vi "top_level.vi"(10 "progress ref":refnum<vi>, 11 "series URL":string) -> (0 "error out":errorcluster, 2 "fetch time":dbl, 3 "seriesInfo":T2)   [LabVIEW 2024]
uses:
  definitions/seriesInfo.ctl
  definitions/issueInfo.ctl
  definitions/creator.ctl
  definitions/character.ctl
  definitions/team.ctl
  definitions/location.ctl
  definitions/concept.ctl
  definitions/thing.ctl
  definitions/storyArc.ctl
  definitions/seriesJSON.ctl
  series_class/series_class.lvclass
  C:/Code/LabVIEW_Projects/applications/ComicVine_API/comic_class/comic_class.lvclass
  series_class/series_class.lvclass/series_class.ctl
  <vilib>/Utility/High Resolution Relative Seconds.vi
  comic_class/comic_class.lvclass
  <vilib>/addons/_JKI.lib/Serialization/JSON/JKI JSON Serialization.lvlib
panel:
  in  "output cluster":T1
  out "issues":T3[](array[typedef])
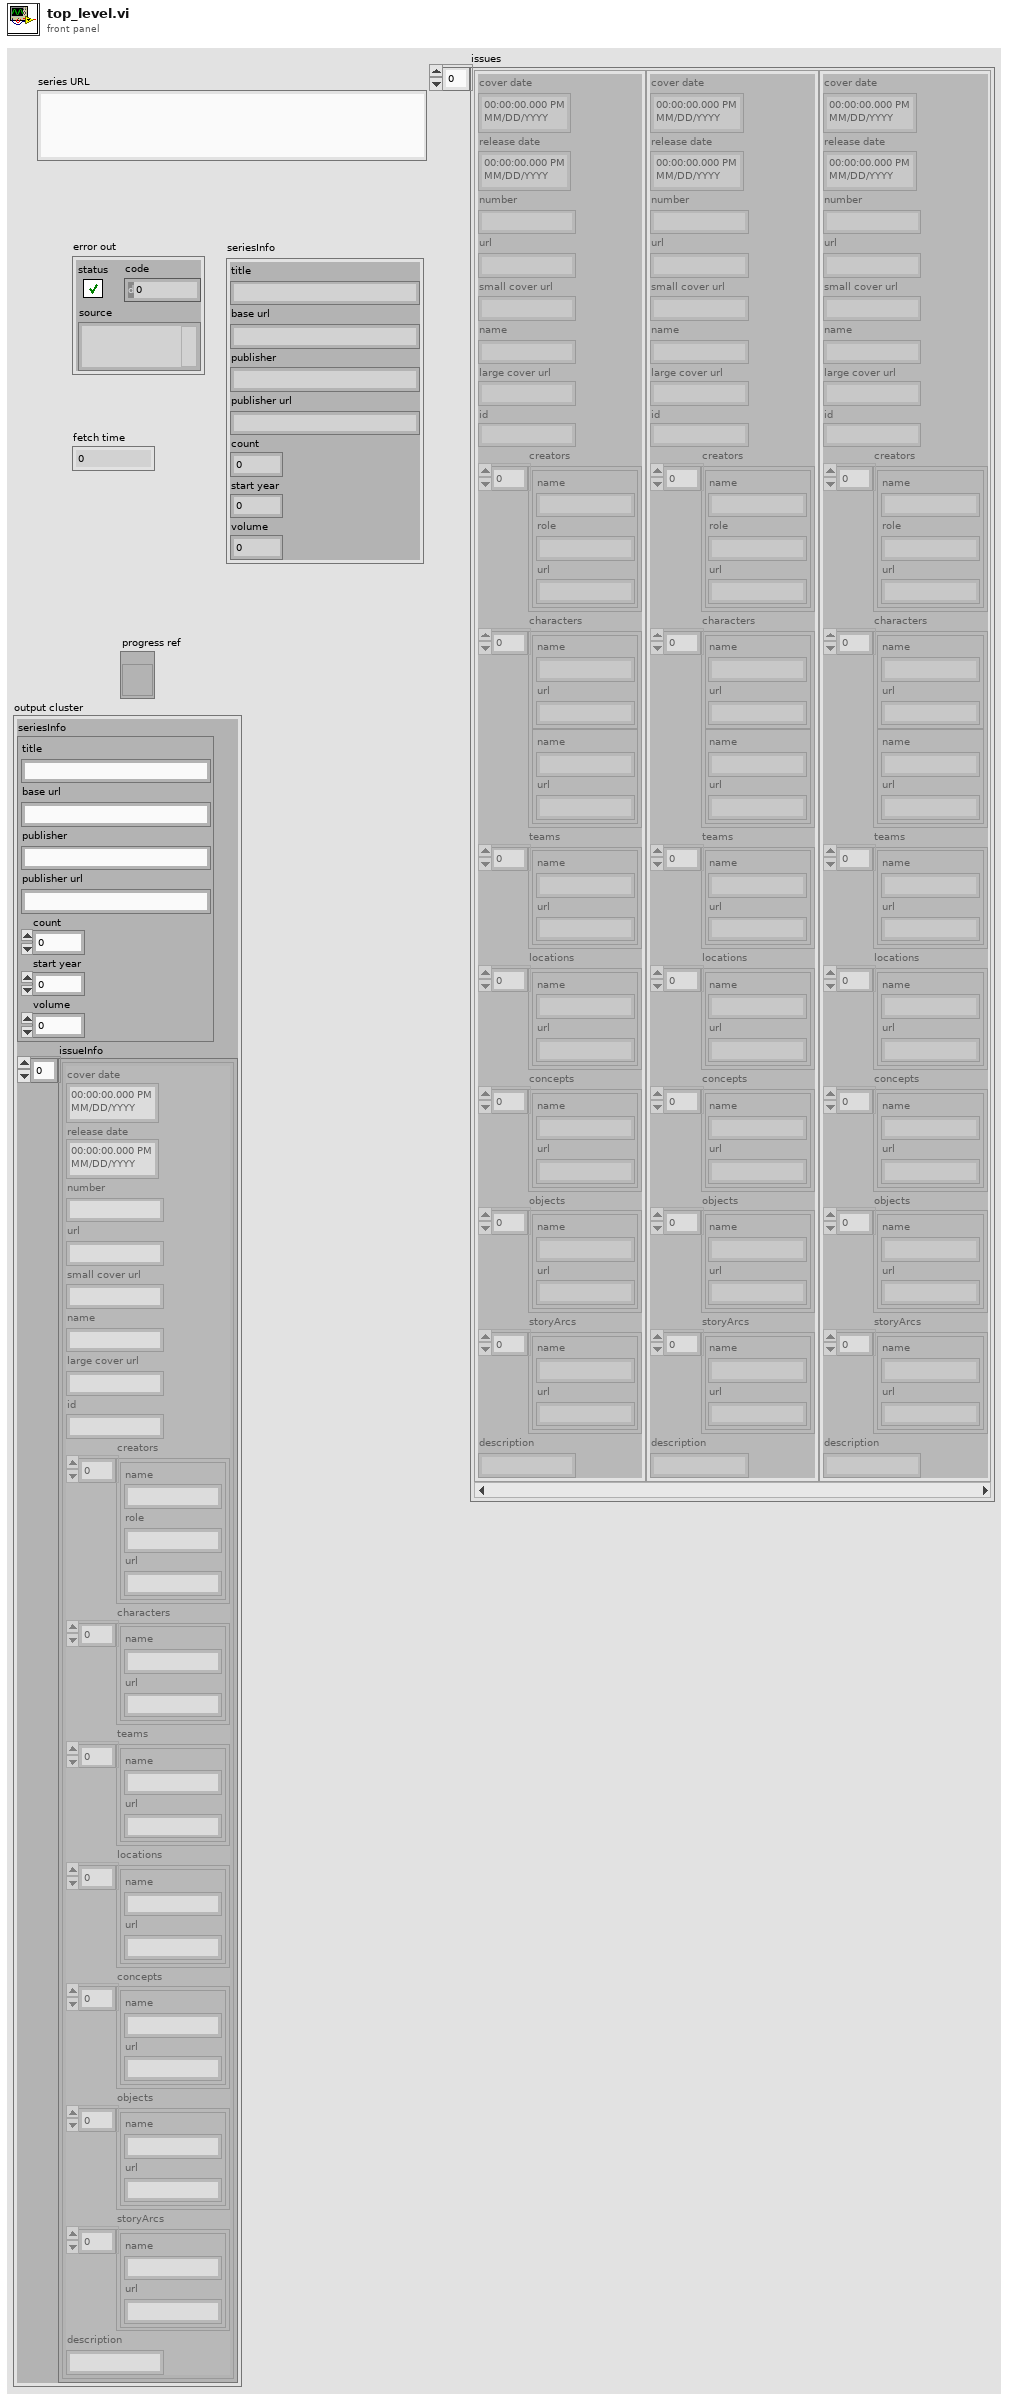
[diagram p1: front panel]
types:
  T1 = typedef "seriesJSON.ctl" = cluster{"seriesInfo":T2, "issueInfo":T3[]}
  T2 = typedef "seriesInfo.ctl" = cluster{"title":string, "base url":string, "publisher":string, "publisher url":string, "count":i32, "start year":i32, "volume":i32}
  T3 = typedef "issueInfo.ctl" = cluster{"cover date":timestamp, "release date":timestamp, "number":string, "url":string, "small cover url":string, "name":string, "large cover url":string, "id":string, "creators":T4[], "characters":T5[], "teams":T6[], "locations":T7[], "concepts":T8[], "objects":T9[], "storyArcs":T10[], "description":string}
  T4 = typedef "creator.ctl" = cluster{"name":string, "role":string, "url":string}
  T5 = typedef "character.ctl" = cluster{"name":string, "url":string}
  T6 = typedef "team.ctl" = cluster{"name":string, "url":string}
  T7 = typedef "location.ctl" = cluster{"name":string, "url":string}
  T8 = typedef "concept.ctl" = cluster{"name":string, "url":string}
  T9 = typedef "thing.ctl" = cluster{"name":string, "url":string}
  T10 = typedef "storyArc.ctl" = cluster{"name":string, "url":string}
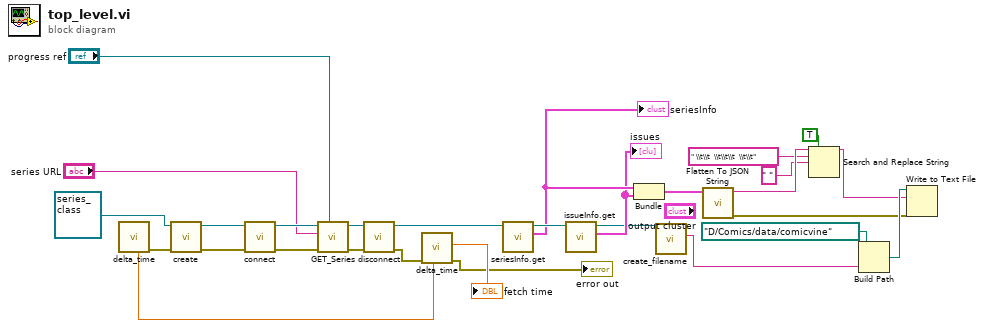
[diagram p0: block diagram]
diagram:
  n1 = call "delta_time.vi"() -> ("error out"=w27:errorcluster, "Time out"=w25:dbl)  [unwired: 9 in, 1 out]
  n2 = call "create.vi"("error in (no error)"=w27, "comic_class in"=refnum<class "series_class.lvclass"> refnum ("series_class.lvclass")) -> ("error out"=w29:errorcluster, "comic_class out"=w28:refnum<class "series_class.lvclass">)  [unwired: 8 in]
  n3 = call-dynamic "connect.vi"("error in (no error)"=w29, "comic_class in"=w28) -> ("error out"=w20:errorcluster, "comic_class out"=w21:refnum<class "series_class.lvclass">)  [unwired: 8 in]
  n4 = call "GET_Series.vi"("progress ref"="progress ref", "error in (no error)"=w20, "series URL"="series URL", "ComicVine_class in"=w21) -> ("error out"=w22:errorcluster, "ComicVine_class out"=w23:refnum<class "series_class.lvclass">)  [unwired: 6 in]
  n5 = call-dynamic "disconnect.vi"("error in (no error)"=w22, "comic_class in"=w23) -> ("error out"=w26:errorcluster, "comic_class out"=w19:refnum<class "series_class.lvclass">)  [unwired: 8 in]
  n6 = call "delta_time.vi"("Time in"=w25, "error in (no error)"=w26) -> ("error out"=→"error out":errorcluster, "Delta Time"=→"fetch time":dbl)  [unwired: 7 in, 1 out]
  n7 = call "seriesInfo.get.vi"("ComicVine_class in"=w19) -> ("seriesInfo"=w15:T2, "ComicVine_class out"=w18:refnum<class "series_class.lvclass">)  [unwired: 9 in]
  "seriesInfo" <- w15
  n8 = call "issueInfo.get.vi"("ComicVine_class in"=w18) -> ("issueInfo"=w14:T3[], "ComicVine_class out"=w9:refnum<class "series_class.lvclass">)  [unwired: 9 in]
  "issues" <- w14
  n9 = Bundle("seriesInfo"=w15, "issueInfo"=w14) -> (w13:cluster{"seriesInfo":T2, "issueInfo":T3[]})  [unwired: 1 in]
  n10 = call "create_filename.vi"("series_class in"=w9) -> ("json filename"=w8:string)  [unwired: 9 in, 1 out]
  n11 = call <vilib>:"Flatten To JSON String.vi"("Variant"=w13) -> ("error out"=w10:errorcluster, "JSON String"=w7:string)  [unwired: 9 in]
  n12 = Search and Replace String(replace all?=TRUE ("replace all? (F)"), input string=w7, search string=" \\t\\t  \\t\\t\\t  \\t\\t", replace string=" " ("replace string (\"\")")) -> (result string=w6:string)  [unwired: 4 in, 3 out]
  n13 = Build Path(base path=path "D:/Comics/data/comicvine", name or relative path=w8) -> (appended path=w11:path)
  n14 = Write to Text File(file (use dialog)=w11, text=w6, error in=w10) -> ()  [unwired: 1 in, 3 out]
